vi "Measure.vi"(6 "error in (no error)":errorcluster, 9 "Yokogawa WT1600 in":refnum<class "Yokogawa WT1600.lvclass">) -> (0 "error out":errorcluster, 2 "Array of Measurement":dbl[](array[numeric]), 3 "Yokogawa WT1600 out":refnum<class "Yokogawa WT1600.lvclass">)   [LabVIEW 2014, in "Generic Power Analyzer.lvlib" / "Yokogawa WT1600.lvlib" / "Yokogawa WT1600.lvclass"]
uses:
  Yokogawa WT1600.lvclass
  Generic Power Analyzer/Generic Power Analyzer.lvclass
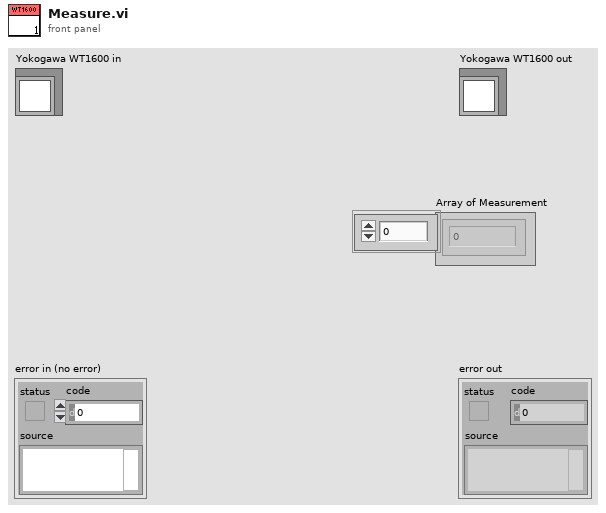
[diagram p1: front panel]
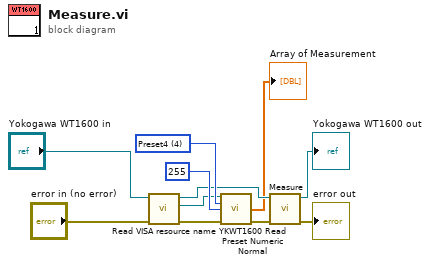
[diagram p0: block diagram]
diagram:
  w8 = u16 4 items=["", "Preset1", "Preset2", "Preset3", "Preset4"] ("Preset (2: Preset 2)")
  n1 = call-dynamic "Read VISA resource name.vi"("error in (no error)"="error in (no error)", "Generic Instrument in"="Yokogawa WT1600 in") -> ("error out"=w2:errorcluster, "VISA resource name"=w4:refnum<visa-resource-name>, "Generic Instrument out"=w5:refnum<class "Yokogawa WT1600.lvclass">)  [unwired: 7 in]
  n2 = call <instrlib>:"YKWT1600 Read Preset Numeric Normal.vi"("VISA session"=w4, "Preset (2: Preset 2)"=w8, "Number of Item (15)"=u16 255, "error in (no error)"=w2) -> ("Measure"=→"Array of Measurement":dbl[], "error out"=w7:errorcluster)  [unwired: 8 in, 2 out]
  n3 = call-parent "Measure.vi"("error in (no error)"=w7, "Generic Power Analyzer in"=w5) -> ("error out"=→"error out":errorcluster, "Generic Power Analyzer out"=→"Yokogawa WT1600 out":refnum<class "Yokogawa WT1600.lvclass">)  [unwired: 5 in, 1 out]
